vi "Get Exported DIDPIDs.vi"(8 "error in (no error)":errorcluster, 10 "GUID":string, 11 "Item Ref in":T4 format="%.0x") -> (0 "error out":errorcluster, 2 "DID/PID":T1 {"DIDPID Array"."Signals"."Byte Order" items=["Little Endian", "Big Endian"]; "DIDPID Array"."Signals"."Data Type" items=["Signed", "Unsigned", "IEEE Float"]}, 3 "Section Ref out":T4 format="%.0x")   [LabVIEW 2013, in "Diagnostics Addon System Explorer.lvlib"]
uses:
  Diagnostics Addon System Explorer.lvlib
  <vilib>/NI Veristand/Custom Device API/Custom Device Item Ref.ctl
  Shared/Exported DIDPIDs Cluster.ctl
  Shared/DIDPID Parameters.ctl
  Shared/DIDPID Signal Parameters.ctl
  Shared/FG Action.ctl
  Shared/Signal Parameters FG.vi
  <vilib>/NI Veristand/Custom Device Tools/Custom Device Utility Library/NI VeriStand - Search for Item by GUID.vi
  Shared/GUID Lookup.vi
  <vilib>/NI Veristand/Custom Device API/NI VeriStand - Get Item Property.vi
  <vilib>/NI Veristand/Custom Device API/Get Item Property (Variant).vi
  <vilib>/NI Veristand/Custom Device API/NI VeriStand - Get Custom Device Channel Data.vi
  <vilib>/NI Veristand/Custom Device Tools/Custom Device Utility Library/Custom Device Utility Library.lvlib
  <vilib>/NI Veristand/Custom Device API/Custom Device API.lvlib
  Shared/Diagnostics Addon Shared.lvlib
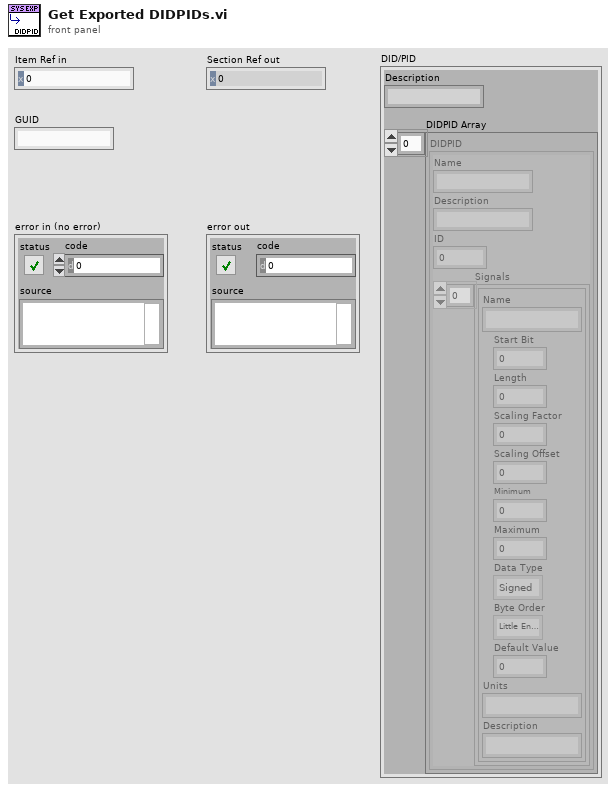
[diagram p1: front panel]
types:
  T1 = typedef "Diagnostics Addon Shared.lvlib/Exported DIDPIDs Cluster.ctl" = cluster{"Description":string, "DIDPID Array":T2[]}
  T2 = typedef "Diagnostics Addon Shared.lvlib/DIDPID Parameters.ctl" = cluster{"Name":string, "Description":string, "ID":u16, "Signals":T3[]}
  T3 = typedef "Diagnostics Addon Shared.lvlib/DIDPID Signal Parameters.ctl" = cluster{"Name":string, "Start Bit":u8, "Length":u8, "Scaling Factor":dbl, "Scaling Offset":dbl, "Minimum":dbl, "Maximum":dbl, "Data Type":u32, "Byte Order":u32, "Default Value":dbl, "Units":string, "Description":string}
  T4 = typedef "Custom Device API.lvlib/Custom Device Item Ref.ctl" = u64
  T5 = typedef "Diagnostics Addon Shared.lvlib/FG Action.ctl" = enum16{"Get", "Set"}
  T6 = typedef "Custom Device API.lvlib/Custom Device Item Info.ctl" = cluster{"Name":string, "Is Channel":bool, "GUID":string, "Is Waveform":bool}
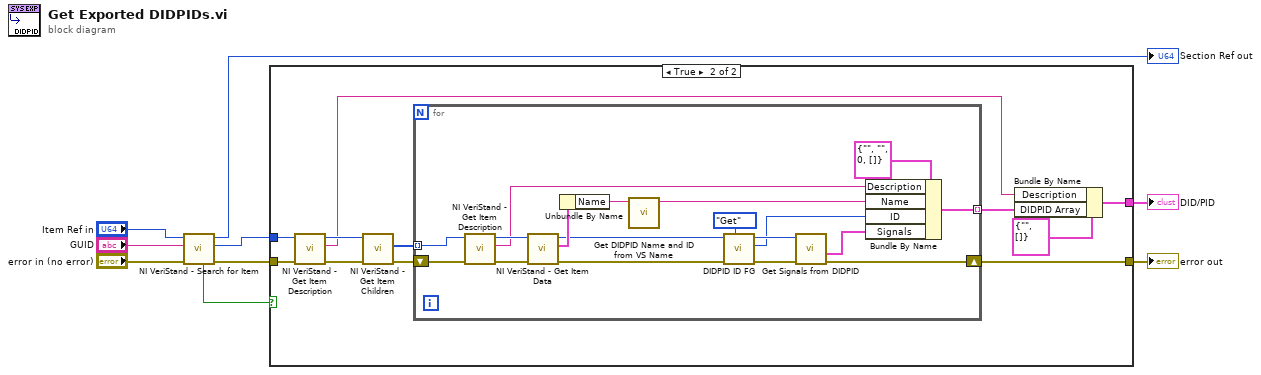
[diagram p0: block diagram]
diagram:
  n1 = call-poly <vilib>:"NI VeriStand - Search for Item.vi"("error in"="error in (no error)", "Item GUID"="GUID", "Section Ref in"="Item Ref in") -> ("error out"=w4:errorcluster, "Item Ref"=w3:T4, "Section Ref out"=→"Section Ref out":T4, "Found"=w2:bool)  [unwired: 5 in]
  n2 = case shown="False" w2 {
    tunnel: [_ w12] -> w1
    tunnel: [w10 w21] -> w5
    tunnel: w4 -> [w10 w16]
    tunnel: w3 -> [_ w18]
    frame False {
    }
    frame True {
      n3 = call <vilib>:"NI VeriStand - Get Item Description.vi"("error in (no error)"=w16, "Item Ref in"=w18) -> ("error out"=w15:errorcluster, "Description"=w13:string, "Item Ref out"=w17:T4)  [unwired: 7 out]
      n4 = call <vilib>:"NI VeriStand - Get Item Children.vi"("error in (no error)"=w15, "Item Ref in"=w17) -> ("error out"=w20:errorcluster, "Child Refs"=w19:T4[])  [unwired: 6 in, 2 out]
      n5 = for {
        tunnel: w19 -> [w36] mode=indexing
        shift-right: [w29] -> w21
        shift-left: w20 -> [w35]
        tunnel: [w25] -> w11 mode=indexing
        n6 = call <vilib>:"NI VeriStand - Get Item Description.vi"("error in (no error)"=w35, "Item Ref in"=w36) -> ("error out"=w38:errorcluster, "Description"=w34:string, "Item Ref out"=w39:T4)  [unwired: 7 out]
        n7 = call <vilib>:"NI VeriStand - Get Item Data.vi"("error in (no error)"=w38, "Item Ref in"=w39) -> ("error out"=w31:errorcluster, "Item Info"=w37:T6, "Item Ref out"=w30:T4)  [unwired: 7 out]
        n8 = Unbundle By Name(w37) -> ("Name"=w23:string)
        n9 = call "Get DIDPID Name and ID from VS Name.vi"("VS PID Name"=w23) -> ("PID Name"=w22:string)  [unwired: 9 in, 1 out]
        n10 = call "DIDPID ID FG.vi"("Action"=FG_Action."Get", "error in (no error)"=w31, "Device Item Ref in"=w30) -> ("error out"=w32:errorcluster, "ID"=w27:u16, "Device Item Ref out"=w33:T4)  [unwired: 6 in]
        n11 = call "Get Signals from DIDPID.vi"("error in (no error)"=w32, "Device Item Ref out"=w33) -> ("error out"=w29:errorcluster, "PID Parameters"=w26:T3[])  [unwired: 6 in, 2 out]
        n12 = Bundle By Name(cluster=T2 {"Name"="", "Description"="", "ID"=0, "Signals"=[]}, "Description"=w34, "Name"=w22, "ID"=w27, "Signals"=w26) -> (w25:T2)
      }
      n13 = Bundle By Name(cluster=T1 {"Description"="", "DIDPID Array"=[]}, "Description"=w13, "DIDPID Array"=w11) -> (w12:T1)
    }
  }
  "error out" <- w5
  "DID/PID" <- w1
